vi "VirtualTestInstrument.vi"(8 "error in (no error)":errorcluster, 10 "Message":T1={"Command"="", "Data"=variant(string ""), "ID"=""}, 11 "RemoteControl":refnum<class "RemoteControl.lvclass">) -> (0 "error out":errorcluster, 2 "processed Message":T1={"Command"="", "Data"=variant(string ""), "ID"=""}, 3 "RemoteControl":refnum<class "RemoteControl.lvclass">)   [LabVIEW 2019, in "RemoteControl.lvclass"]
uses:
  RemoteControl.lvclass
  Typedefs/Message--Cluster.ctl
  RemoteControl.lvclass/RemoteControl.ctl
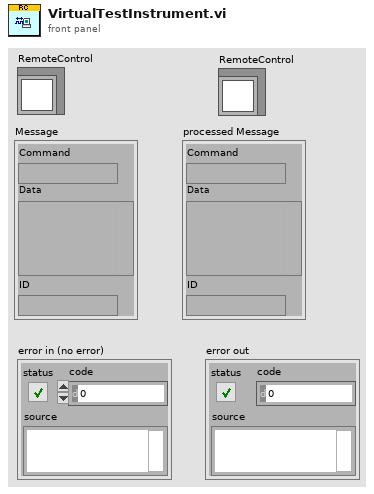
[diagram p1: front panel]
types:
  T1 = typedef "RemoteControl.lvclass/Message--Cluster.ctl" = cluster{"Command":string, "Data":variant, "ID":string}
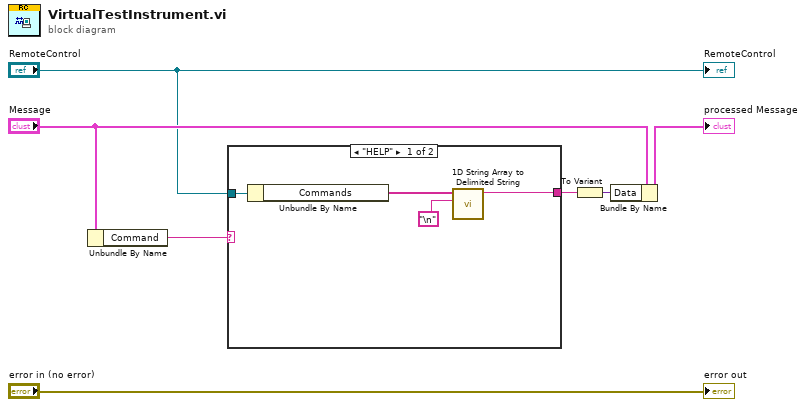
[diagram p0: block diagram]
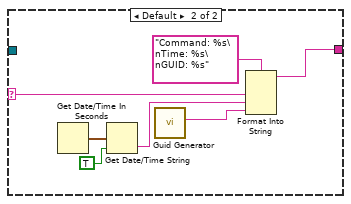
[diagram p2: hidden frame]
diagram:
  n1 = Unbundle By Name("Message") -> ("Command"=w2:string)
  n2 = case shown="\"HELP\"" w2 {
    selector: w2 -> [_ w13]
    tunnel: [w9 w12] -> w3
    tunnel: "RemoteControl" -> [w11 _]
    frame "HELP" {
      n3 = Unbundle By Name(w11) -> ("Commands"=w10:string[])
      n4 = call <vilib>:"1D String Array to Delimited String.vi"("delimiter"="\n", "string array"=w10) -> ("delimited string"=w9:string)  [unwired: 9 in]
    }
    frame Default {
      n5 = Get Date/Time In Seconds() -> (seconds since 1Jan1904=w17:timestamp)
      n6 = Get Date/Time String(seconds (now)=w17, want seconds? (F)=TRUE) -> (time string=w14:string)  [unwired: 1 in, 1 out]
      n7 = call <vilib>:"Guid Generator.vi"() -> ("GUID"=w15:string)  [unwired: 10 in, 1 out]
      n8 = Format Into String(format string="Command: %s\nTime: %s\nGUID: %s", w13, w14, w15) -> (resulting string=w12:string)  [unwired: 2 in, 1 out]
    }
  }
  n9 = To Variant(anything=w3) -> (Variant=w1:variant)
  n10 = Bundle By Name(cluster="Message", "Data"=w1) -> (→"processed Message":T1)
  "error out" <- "error in (no error)"
  "RemoteControl" <- "RemoteControl"
